vi "Clear-object.vi"(8 "error in (no error)":errorcluster, 11 "Errors in":T1) -> (0 "error out":errorcluster, 3 "Errors out":T1)   [LabVIEW 2013, in "CameraVision.lvlib" / "CV-Errors.lvclass"]
uses:
  CV-Errors.lvclass
  Object-reference.ctl
  CV-Errors.lvclass/CV-Errors.ctl
  Read Error event.vi
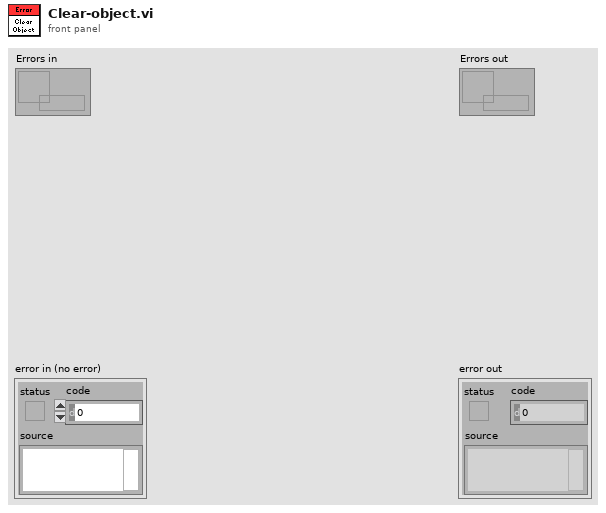
[diagram p1: front panel]
types:
  T1 = typedef "CameraVision.lvlib/CV-Errors.lvclass/Object-reference.ctl" = refnum<data-value>
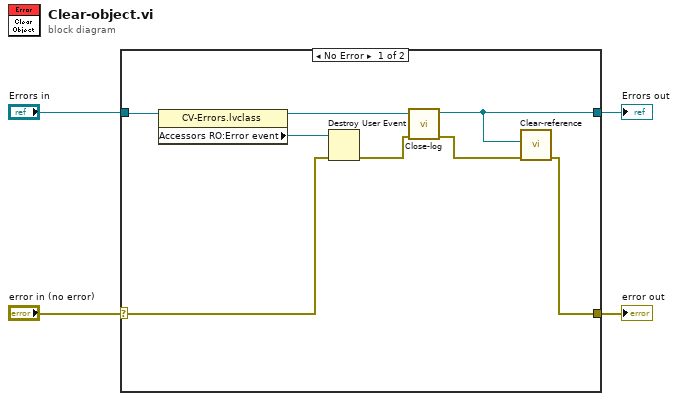
[diagram p0: block diagram]
diagram:
  n1 = case shown="No Error" "error in (no error)" {
    selector: "error in (no error)" -> [w8 w13]
    tunnel: [w10 w13] -> w3
    tunnel: [w12 w14] -> w1
    tunnel: "Errors in" -> [w7 w14]
    frame No Error {
      n2 = property class="CV-Errors.lvclass"(reference=w7) -> (reference out=w5:T1, "Accessors RO:Error event"=w6:refnum<user-event>)  [unwired: 1 in, 1 out]
      n3 = Destroy User Event(user event=w6, error in=w8) -> (error out=w9:errorcluster)
      n4 = call "Close-log.vi"("error in (no error)"=w9, "Errors in"=w5) -> ("error out"=w11:errorcluster, "Errors out"=w12:T1)  [unwired: 8 in]
      n5 = call "Clear-reference.vi"("error in (no error)"=w11, "Errors reference"=w12) -> ("error out"=w10:errorcluster)  [unwired: 8 in, 1 out]
    }
    frame Error {
    }
  }
  "error out" <- w3
  "Errors out" <- w1
